vi "Table_SetFontSize.vi"(8 "error in":errorcluster, 9 "Listbox Settings":T1, 10 "Array Sizes":i32[](array[numeric]), 11 "Listbox Ref":refnum<vi>) -> (0 "error out":errorcluster, 3 "Listbox Ref Out":refnum<vi>)   [LabVIEW 2012, in "TableSupportLib.lvlib"]
uses:
  TableSupportLib.lvlib
  Table_ListboxSettings.ctl
  <vilib>/Utility/miscctls.llb/LVRowAndColumnTypeDef.ctl
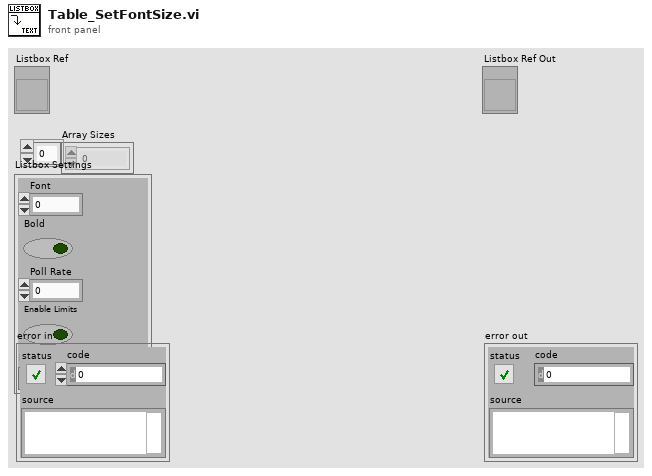
[diagram p1: front panel]
types:
  T1 = typedef "TableSupportLib.lvlib/Table_ListboxSettings.ctl" = cluster{"Font":u32, "Bold":bool, "Poll Rate":u32, "Enable Limits":bool, "Path":path}
  T2 = typedef "LVRowAndColumnTypeDef.ctl" = cluster{"Row":i32, "Column":i32}
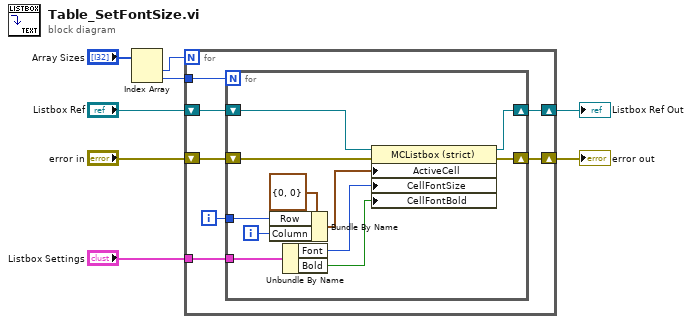
[diagram p0: block diagram]
diagram:
  n1 = Index Array(array="Array Sizes") -> (element #1=w8:i32, element #2=w7:i32)  [unwired: 2 in]
  n2 = for {
    N: w8 -> [_]
    tunnel: w7 -> [w13]
    tunnel: "Listbox Settings" -> [w12]
    shift-right: [w11] -> w3
    shift-left: "error in" -> [w10]
    shift-right: [w9] -> w1
    shift-left: "Listbox Ref" -> [w14]
    i -> [w15]
    n3 = for {
      N: w13 -> [_]
      tunnel: w15 -> [w23]
      tunnel: w12 -> [w21]
      shift-right: [w18] -> w11
      shift-left: w10 -> [w17]
      shift-right: [w16] -> w9
      shift-left: w14 -> [w22]
      i -> [w26]
      n4 = Bundle By Name(cluster=T2 {"Row"=0, "Column"=0} ("Active Cell:Active Cell"), "Row"=w23, "Column"=w26) -> (w24:T2)
      n5 = Unbundle By Name(w21) -> ("Font"=w20:u32, "Bold"=w19:bool)
      n6 = property class="MCListbox (strict)"(reference=w22, error in=w17, "ActiveCell"=w24, "CellFontSize"=w20, "CellFontBold"=w19) -> (reference out=w16:refnum<vi>, error out=w18:errorcluster)
    }
  }
  "error out" <- w3
  "Listbox Ref Out" <- w1
